vi "Data Lookup Table Get Signals (Range).vi"(8 "error in (no error)":errorcluster, 10 "Direct Access":cluster{"Offset":u32, "Length":u32}, 11 "Data Ref":T1) -> (0 "error out":errorcluster {"code" min=0 max=0}, 2 "Signals":dbl[](array[numeric]), 3 "Data Ref out":T1)   [LabVIEW 2015, in "J1939 Addon Engine.lvlib"]
uses:
  J1939 Addon Engine.lvlib
  Types/Data Lookup Table Reference.ctl
  Types/Datatable Lookup DVR.ctl
  Types/Data Lookup Table Action.ctl
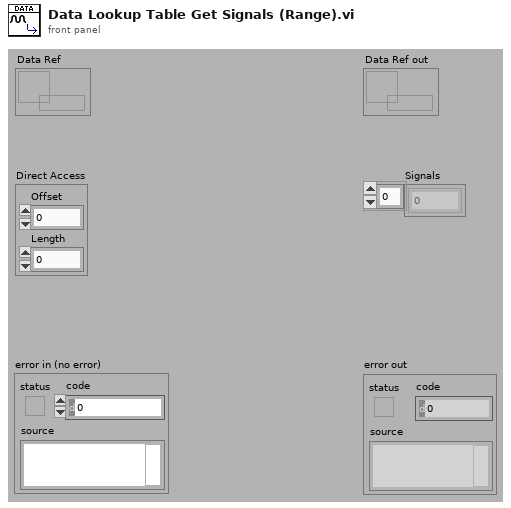
[diagram p1: front panel]
types:
  T1 = typedef "J1939 Addon Engine.lvlib/Data Lookup Table Reference.ctl" = refnum<data-value>
  T2 = typedef "J1939 Addon Engine.lvlib/Data Lookup Table Action.ctl" = enum16{"Get All", "Set All", "Set Frame", "Get Frame", "Set Range", "Get Range"}
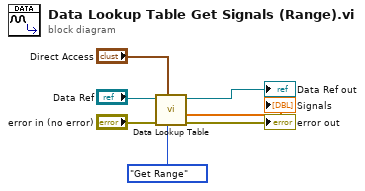
[diagram p0: block diagram]
diagram:
  n1 = call "Data Lookup Table.vi"("command"=Data_Lookup_Table_Action."Get Range", "Direct Access"="Direct Access", "error in (no error)"="error in (no error)", "Data Ref"="Data Ref") -> ("error out"=→"error out":errorcluster, "Signals Out"=→"Signals":dbl[], "Data Ref out"=→"Data Ref out":T1)  [unwired: 5 in]
